vi "Build_Asylum_WriteValue.vi"(8 "error in (no error)":errorcluster, 10 "value":dbl, 11 "parameterName":string) -> (0 "error out":errorcluster, 3 "Command":string)   [LabVIEW 2019]
uses:
  <vilib>/Utility/error.llb/whitespace.ctl
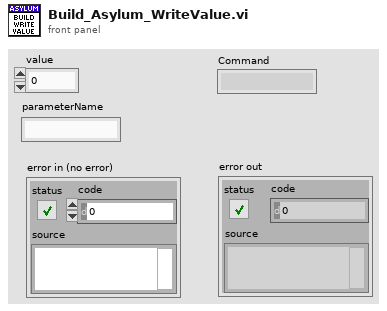
[diagram p1: front panel]
types:
  T1 = typedef "whitespace.ctl" = u16
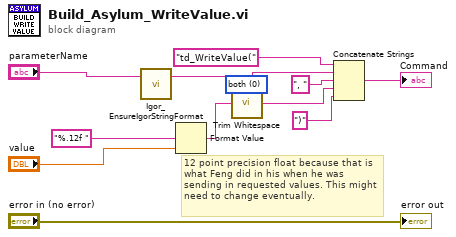
[diagram p0: block diagram]
diagram:
  w2 = T1 0 items=["both", "start of string", "end of string"] ("location (both)")
  # "12 point precision float because that is what Feng did in his when he was sending in requested values. This might need to change eventually."
  n1 = call <userlib>:"Igor_EnsureIgorStringFormat.vi"("Value"="parameterName") -> ("Value"=w11:string)  [unwired: 2 in]
  n2 = Format Value(format string="%.12f ", value (0)="value") -> (output string=w4:string)  [unwired: 1 in]
  n3 = call <vilib>:"Trim Whitespace.vi"("string"=w4, "location (both)"=w2) -> ("trimmed string"=w3:string)
  n4 = Concatenate Strings("td_WriteValue(" ("string"), w11, ", " ("string"), w3, ")" ("string")) -> (→"Command":string)
  "error out" <- "error in (no error)"
